vi "config.vi"(8 "error in (no error)":errorcluster, 11 "Impedancia":string(combo)="0") -> (0 "error out":errorcluster)   [LabVIEW 2019, in "DS360_GPIB.lvlib"]
uses:
  DS360_GPIB.lvlib
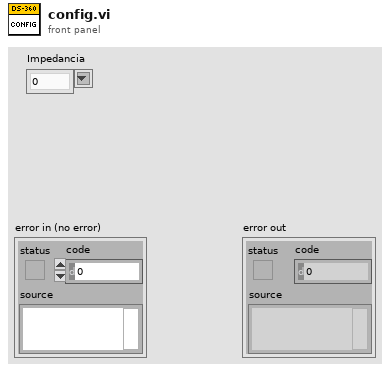
[diagram p1: front panel]
types:
  T1 = cluster{"error":bool, "code":i32, "source":string}
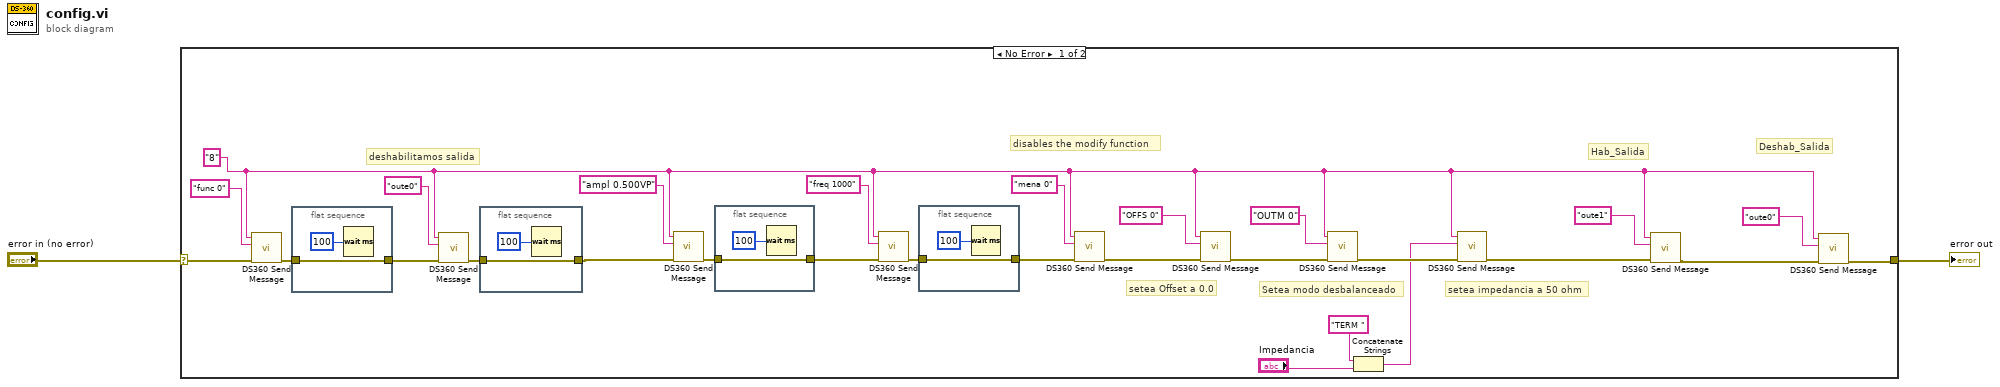
[diagram p0: block diagram]
diagram:
  n1 = case shown="No Error" "error in (no error)" {
    selector: "error in (no error)" -> [w25 w39]
    tunnel: [w13 w39] -> w1
    frame No Error {
      w4 = "8" ("write buffer")
      # "setea impedancia a 50 ohm"
      # "Setea modo desbalanceado"
      # "setea Offset a 0.0"
      # "Deshab_Salida"
      # "Hab_Salida"
      # "disables the modify function"
      # "deshabilitamos salida"
      n2 = call <instrlib>:"DS360 Send Message.vi"("address string"=w4, "write buffer"="func 0", "error in"=w25) -> ("error out"=w28:T1)  [unwired: 3 in, 3 out]
      n3 = flat-sequence {
        tunnel: w28 -> [w38]
        tunnel: [w38] -> w27
        frame #0 {
          n4 = Wait (ms)(milliseconds to wait=u32 100) -> ()  [unwired: 1 out]
        }
      }
      n5 = call <instrlib>:"DS360 Send Message.vi"("address string"=w4, "write buffer"="oute0", "error in"=w27) -> ("error out"=w26:T1)  [unwired: 3 in, 3 out]
      n6 = flat-sequence {
        tunnel: w26 -> [w36]
        tunnel: [w36] -> w17
        frame #0 {
          n7 = Wait (ms)(milliseconds to wait=u32 100) -> ()  [unwired: 1 out]
        }
      }
      n8 = call <instrlib>:"DS360 Send Message.vi"("address string"=w4, "write buffer"="ampl 0.500VP", "error in"=w17) -> ("error out"=w21:T1)  [unwired: 3 in, 3 out]
      n9 = flat-sequence {
        tunnel: w21 -> [w34]
        tunnel: [w34] -> w20
        frame #0 {
          n10 = Wait (ms)(milliseconds to wait=u32 100) -> ()  [unwired: 1 out]
        }
      }
      n11 = call <instrlib>:"DS360 Send Message.vi"("address string"=w4, "write buffer"="freq 1000", "error in"=w20) -> ("error out"=w19:T1)  [unwired: 3 in, 3 out]
      n12 = flat-sequence {
        tunnel: w19 -> [w32]
        tunnel: [w32] -> w18
        frame #0 {
          n13 = Wait (ms)(milliseconds to wait=u32 100) -> ()  [unwired: 1 out]
        }
      }
      n14 = call <instrlib>:"DS360 Send Message.vi"("address string"=w4, "write buffer"="mena 0", "error in"=w18) -> ("error out"=w5:T1)  [unwired: 3 in, 3 out]
      n15 = call <instrlib>:"DS360 Send Message.vi"("address string"=w4, "write buffer"="OFFS 0", "error in"=w5) -> ("error out"=w11:T1)  [unwired: 3 in, 3 out]
      n16 = call <instrlib>:"DS360 Send Message.vi"("address string"=w4, "write buffer"="OUTM 0", "error in"=w11) -> ("error out"=w10:T1)  [unwired: 3 in, 3 out]
      n17 = Concatenate Strings("TERM " ("write buffer"), "Impedancia") -> (w6:string)
      n18 = call <instrlib>:"DS360 Send Message.vi"("address string"=w4, "write buffer"=w6, "error in"=w10) -> ("error out"=w3:T1)  [unwired: 3 in, 3 out]
      n19 = call <instrlib>:"DS360 Send Message.vi"("address string"=w4, "write buffer"="oute1", "error in"=w3) -> ("error out"=w14:T1)  [unwired: 3 in, 3 out]
      n20 = call <instrlib>:"DS360 Send Message.vi"("address string"=w4, "write buffer"="oute0", "error in"=w14) -> ("error out"=w13:T1)  [unwired: 3 in, 3 out]
    }
    frame Error {
    }
  }
  "error out" <- w1
